vi "BRig_RT__Case_Exp__generic__incrementCountTilThreshold.vi"(11 "input_dataCurrent":u16[](array[numeric])) -> (3 "output_dataCurrent":u16[](array[numeric]), 5 "output_underThreshold":bool)   [LabVIEW 2014]
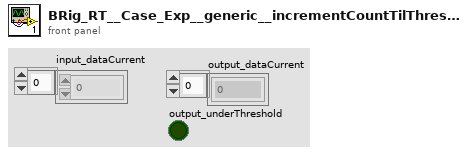
[diagram p1: front panel]
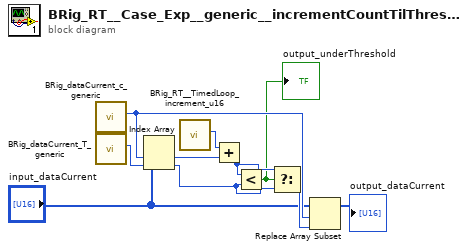
[diagram p0: block diagram]
diagram:
  n1 = call "BRig_dataCurrent_c_generic.vi"() -> ("output_count_generic"=w9:i32)  [unwired: 11 in]
  n2 = call "BRig_dataCurrent_T_generic.vi"() -> ("output_T_generic"=w10:i32)  [unwired: 11 in]
  n3 = Index Array(array="input_dataCurrent", index #1=w9, index #2=w10) -> (element #1=w4:u16, element #2=w7:u16)
  n4 = call "BRig_RT__TimedLoop_increment_u16.vi"() -> ("output_increment__u16"=w3:u16)  [unwired: 11 in]
  n5 = Add(x=w3, y=w4) -> (x+y=w8:u16)
  n6 = Less?(x=w8, y=w7) -> (x < y?=w5:bool)
  "output_underThreshold" <- w5
  n7 = Select(t=w8, s=w5, f=w7) -> (s? t:f=w6:u16)
  n8 = Replace Array Subset(array="input_dataCurrent", new element=w6, index=w9) -> (→"output_dataCurrent":u16[])
